vi "Python_ManageScanPattern.vi"() -> ()   [LabVIEW 2018]
panel:
  out "All signals":dbl[][](graph)
  in  "AO\nrow: rest, illumination\ncol: X, Y, Z":dbl[][](array[numeric])=[[5.0, 5.0, 0.0, 0.0, 0.0, 1.0], [-0.2, 2.9, 0.0, 0.0, 0.0, 0.0]]
  in  "Timing":T1={"Size (pix)"=1024, "Exposure (s)"=0.1, "Slice (s)"=0.0, "Series (s)"=0.0} {"Size (pix)" items=["2048"=2048, "1024"=1024, "512"=512, "256"=256]}
  in  "Beam":T2={"n spirals"=5, "A spiral (V)"=0.8, "sigma"=2.0, "SLIM"=TRUE}
  in  "DAQ":T3={"Ramp time (s)"=0.01, "DAQ rate (Hz)"=10000.0, "X0 (V)"=5.0, "Xc (V)"=-0.2, "Y0 (V)"=5.0, "Yc (V)"=2.9, "Z0 (V)"=0.0, "Zc (V)"=0.0}
  in  "Stack":T4={"LED (V)"=1.0, "#z steps"=1, "z step (V)"=1.0, "UV (%)"=0.2} {"UV (%)" format="%#_13g"}
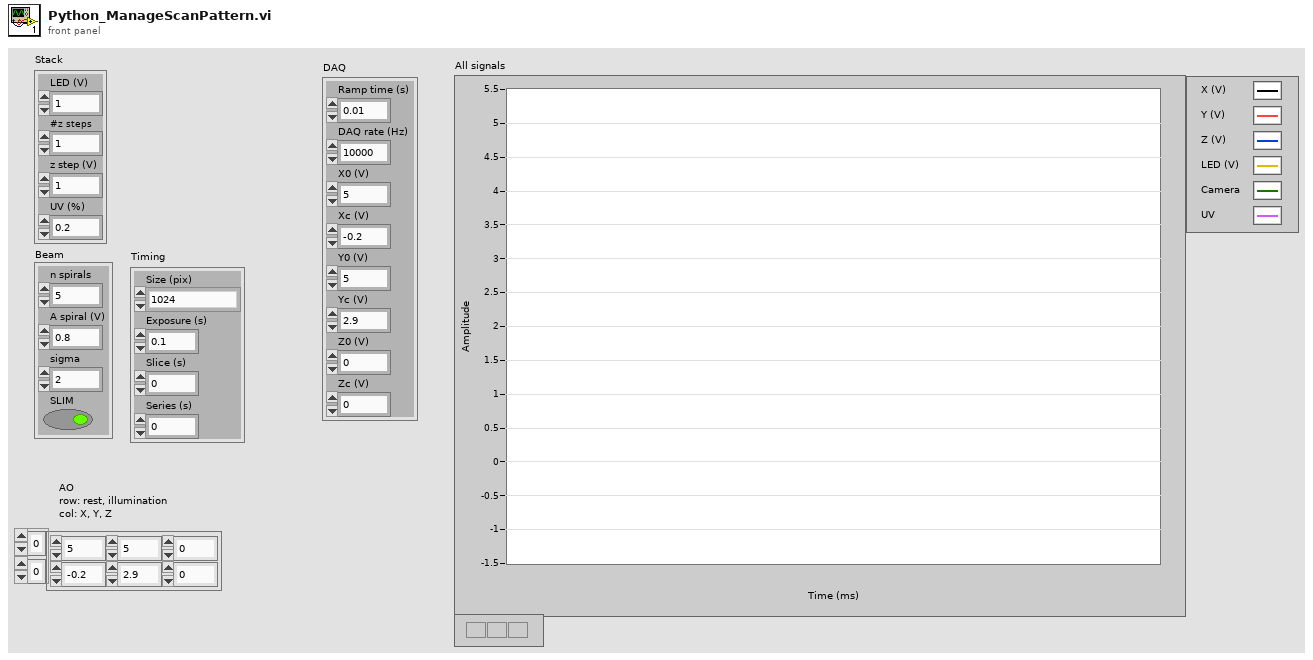
[diagram p1: front panel]
types:
  T1 = cluster{"Size (pix)":u16, "Exposure (s)":dbl, "Slice (s)":dbl, "Series (s)":dbl}
  T2 = cluster{"n spirals":u32, "A spiral (V)":dbl, "sigma":dbl, "SLIM":bool}
  T3 = cluster{"Ramp time (s)":dbl, "DAQ rate (Hz)":dbl, "X0 (V)":dbl, "Xc (V)":dbl, "Y0 (V)":dbl, "Yc (V)":dbl, "Z0 (V)":dbl, "Zc (V)":dbl}
  T4 = cluster{"LED (V)":dbl, "#z steps":i64, "z step (V)":dbl, "UV (%)":dbl}
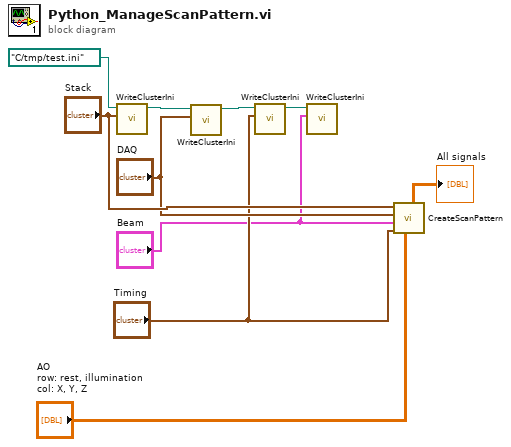
[diagram p0: block diagram]
diagram:
  n1 = call "WriteClusterIni.vi"("cluster variant"="Stack", "configuration file path"=path "C:/tmp/test.ini") -> ("file path out"=w7:path)  [unwired: 8 in, 1 out]
  n2 = call "WriteClusterIni.vi"("cluster variant"="DAQ", "configuration file path"=w7) -> ("file path out"=w5:path)  [unwired: 8 in, 1 out]
  n3 = call "WriteClusterIni.vi"("cluster variant"="Timing", "configuration file path"=w5) -> ("file path out"=w4:path)  [unwired: 8 in, 1 out]
  n4 = call "WriteClusterIni.vi"("cluster variant"="Beam", "configuration file path"=w4) -> ()  [unwired: 8 in, 2 out]
  n5 = call "CreateScanPattern.vi"("AO\nrow: rest, illumination\ncol: X, Y, Z"="AO\nrow: rest, illumination\ncol: X, Y, Z", "Timing"="Timing", "Beam"="Beam", "DAQ"="DAQ", "Stack"="Stack") -> ("All signals"=→"All signals":dbl[][])  [unwired: 3 in, 3 out]
